vi "Clear Button States.vi"(8 "error in (no error)":errorcluster, 11 "Control in":refnum<class "Control.lvclass">) -> (0 "error out":errorcluster, 3 "Control out":refnum<class "Control.lvclass">)   [LabVIEW 2013, in "uitools_Control.lvlib" / "Control.lvclass"]
uses:
  Control.lvclass
  <userlib>/BitMan/BitMap class/BitMap.lvclass
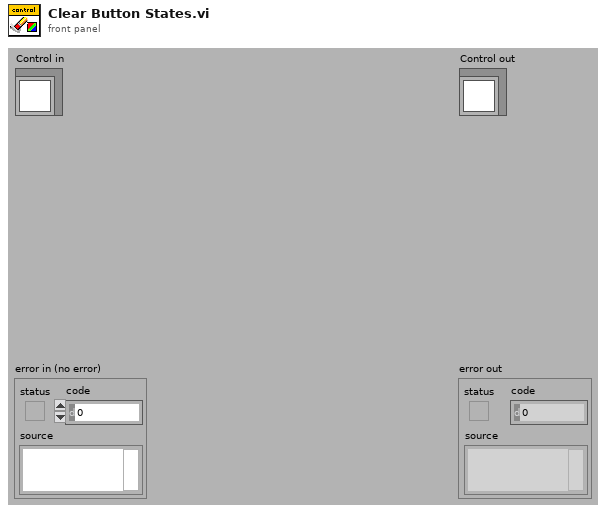
[diagram p1: front panel]
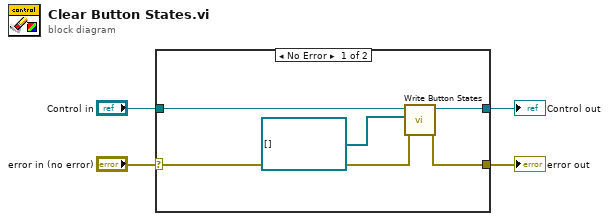
[diagram p0: block diagram]
diagram:
  n1 = case shown="No Error" "error in (no error)" {
    selector: "error in (no error)" -> [w6 w11]
    tunnel: [w5 w11] -> w3
    tunnel: [w8 w10] -> w1
    tunnel: "Control in" -> [w9 w10]
    frame No Error {
      n2 = call-dynamic "Write Button States.vi"("error in (no error)"=w6, "Button States"=refnum<class "BitMap.lvclass">[] [], "Control in"=w9) -> ("error out"=w5:errorcluster, "Control out"=w8:refnum<class "Control.lvclass">)  [unwired: 7 out]
    }
    frame Error {
    }
  }
  "error out" <- w3
  "Control out" <- w1
